vi "Switch to Bank 0.vi"(8 "error in (no error)":errorcluster, 11 "Chip Address (A2 A1 A0)":T2 max=7) -> (0 "error out":errorcluster, 3 "SPI Command":T1)   [LabVIEW 2014, in "MCP23S17.lvlib"]
doc: "Switches the IOCON.BANK to 0 from 1. This process will mess up two of the interrupt control registers if IOCON.BANK already is 0."
uses:
  MCP23S17.lvlib
  Chip Address.ctl
  SPI Command.ctl
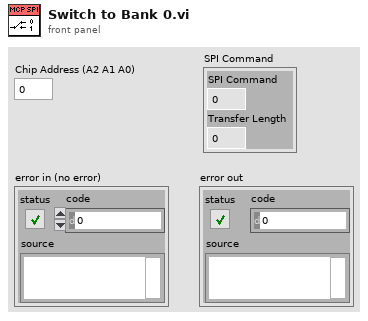
[diagram p1: front panel]
types:
  T1 = typedef "MCP23S17.lvlib/SPI Command.ctl" = cluster{"SPI Command":u32, "Transfer Length":u8}
  T2 = typedef "MCP23S17.lvlib/Chip Address.ctl" = u8
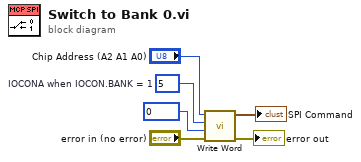
[diagram p0: block diagram]
diagram:
  w2 = u8 5  # IOCONA when IOCON.BANK = 1
  n1 = call "Write Word.vi"("error in (no error)"="error in (no error)", "Value"=u16 0, "Reg Address"=w2, "Chip Address (A2 A1 A0)"="Chip Address (A2 A1 A0)") -> ("error out"=→"error out":errorcluster, "SPI Command"=→"SPI Command":T1)  [unwired: 6 in]
